vi "PWM_Lenkung_Array.vi"(7 "schräg links":dbl, 8 "schräg rechts":dbl, 9 "vorne links":dbl, 10 "vorne rechts":dbl) -> (0 "16 IR true":bool, 2 "PWM Lenkung":dbl, 3 "Linefollow_Array":bool[](array[boolean]))   [LabVIEW 2016]
doc: "VI berrechnet Abweichung des Linearray zur Mittellinie\n05.04.17_Tloe"
uses:
  <vilib>/myRIO/Instrument Drivers/Onboard IO/DIO/typedefs/DIO Reference.ctl
  <vilib>/myRIO/Common/Instrument Driver Framework/Utilities/typedefs/myRIO Generic Hardware Reference.ctl
  <vilib>/myRIO/Common/Instrument Driver Framework/Utilities/typedefs/Hardware Version Enum.ctl
  <vilib>/myRIO/Common/Instrument Driver Framework/Utilities/typedefs/myRIO v1.0 Reference.ctl
  <vilib>/myRIO/Common/Instrument Driver Framework/Utilities/typedefs/Generic FPGA Reference.ctl
  <vilib>/myRIO/Common/Instrument Driver Framework/myRIO v1.0/DIO/typedefs/DIO Channels List.ctl
  <vilib>/myRIO/Common/Instrument Driver Framework/myRIO v1.0/DIO/typedefs/DIO Channels Enum.ctl
  <vilib>/userdefined/High Color/nirio_resource_hc.ctl
  <vilib>/myRIO/Common/Instrument Driver Framework/Utilities/vis/Is FPGA Ref Available.vi
  <vilib>/myRIO/Common/Instrument Driver Framework/myRIO v1.0/DIO/vis/myRIO v1.1 Open DIO.vi
  <vilib>/myRIO/Instrument Drivers/Onboard IO/DIO/vis/Read.vi
  <vilib>/myRIO/Common/Instrument Driver Framework/Utilities/vis/Validate Channels.vi
  <vilib>/myRIO/Common/Instrument Driver Framework/myRIO v1.0/DIO/vis/myRIO v1.0 Reserve DIO.vi
  <vilib>/myRIO/Common/Instrument Driver Framework/myRIO v1.0/Resource Manager/vis/myRIO v1.0 Reserve Channel List.vi
  <vilib>/myRIO/Common/Instrument Driver Framework/myRIO v1.0/DIO/vis/myRIO v1.0 Build MUX Configuration DIO.vi
  <vilib>/myRIO/Common/Instrument Driver Framework/myRIO v1.0/Resource Manager/vis/myRIO v1.0 Reserve Channel.vi
  <vilib>/myRIO/Common/Instrument Driver Framework/myRIO v1.0/Resource Manager/vis/myRIO v1.0 Unreserve Channel.vi
  <vilib>/myRIO/Common/Instrument Driver Framework/myRIO v1.0/Resource Manager/vis/myRIO v1.0 Create Configuration List.vi
  <vilib>/myRIO/Common/Instrument Driver Framework/myRIO v1.0/Resource Manager/vis/myRIO v1.0 Build Mutex Name.vi
  <vilib>/Utility/VariantDataType/GetNumericInfo.vi
  <vilib>/Utility/error.llb/Error Cluster From Error Code.vi
  <vilib>/myRIO/Common/Instrument Driver Framework/myRIO v1.0/myRIO v1.1 Open.vi
  <vilib>/myRIO/Common/Instrument Driver Framework/Utilities/vis/IO Manager.vi
  <vilib>/myRIO/Common/Instrument Driver Framework/Utilities/vis/Configuration Manager.vi
  <vilib>/myRIO/Common/Instrument Driver Framework/myRIO v1.0/Resource Manager/vis/myRIO v1.0 Configure IO.vi
  <vilib>/myRIO/Common/Instrument Driver Framework/myRIO v1.0/myRIO v1.0 Close.vi
  <vilib>/myRIO/Common/Instrument Driver Framework/myRIO v1.0/DIO/vis/myRIO v1.0 Read DIO.vi
  <vilib>/addons/control/pid/pid.llb/PID (DBL).vi
  <vilib>/myRIO/Express VI/Onboard IO/DI/DI Express VI.xnode
  <vilib>/myRIO/Instrument Drivers/Onboard IO/DIO/vis/myRIO DIO Open.xnode
  <vilib>/myRIO/Instrument Drivers/Onboard IO/DIO/DIO.lvlib
  <vilib>/addons/control/pid/NI_PID_pid.lvlib
panel:
  in  "PID Lenkung IR":T1={"proportional gain (Kc)"=0.5, "integral time (Ti, min)"=0.0, "derivative time (Td, min)"=0.002}
  in  "PID Array":T1={"proportional gain (Kc)"=0.8, "integral time (Ti, min)"=0.08, "derivative time (Td, min)"=0.32}
  in  "Sensorarray\nZusatzwerte":dbl[](array[numeric])=[8.0, 7.0, 6.0, 5.0, 4.0, 3.0, 2.0, 1.0, -1.0, -2.0, -3.0, -4.0, -5.0, -6.0, -7.0, -8.0]
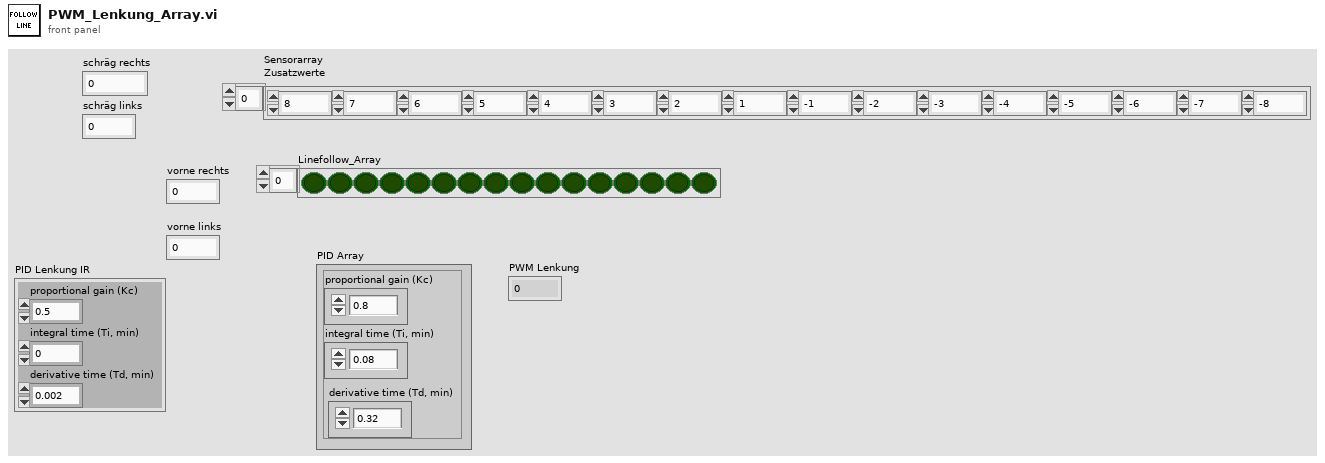
[diagram p1: front panel]
types:
  T1 = cluster{"proportional gain (Kc)":dbl, "integral time (Ti, min)":dbl, "derivative time (Td, min)":dbl}
  T2 = cluster{"A/DIO0 (Pin 11)":bool, "A/DIO1 (Pin 13)":bool, "A/DIO2 (Pin 15)":bool, "A/DIO3 (Pin 17)":bool, "A/DIO4 (Pin 19)":bool, "A/DIO5 (Pin 21)":bool, "A/DIO6 (Pin 23)":bool, "A/DIO7 (Pin 25)":bool, "B/DIO7 (Pin 25)":bool, "B/DIO6 (Pin 23)":bool, "B/DIO5 (Pin 21)":bool, "B/DIO3 (Pin 17)":bool, "B/DIO4 (Pin 19)":bool, "B/DIO2 (Pin 15)":bool, "B/DIO1 (Pin 13)":bool, "B/DIO12 (Pin 22)":bool}
  T3 = cluster{"A/DIO0 (Pin 11)":i16, "A/DIO1 (Pin 13)":i16, "A/DIO2 (Pin 15)":i16, "A/DIO3 (Pin 17)":i16, "A/DIO4 (Pin 19)":i16, "A/DIO5 (Pin 21)":i16, "A/DIO6 (Pin 23)":i16, "A/DIO7 (Pin 25)":i16, "B/DIO7 (Pin 25)":i16, "B/DIO6 (Pin 23)":i16, "B/DIO5 (Pin 21)":i16, "B/DIO3 (Pin 17)":i16, "B/DIO4 (Pin 19)":i16, "B/DIO2 (Pin 15)":i16, "B/DIO1 (Pin 13)":i16, "B/DIO12 (Pin 22)":i16}
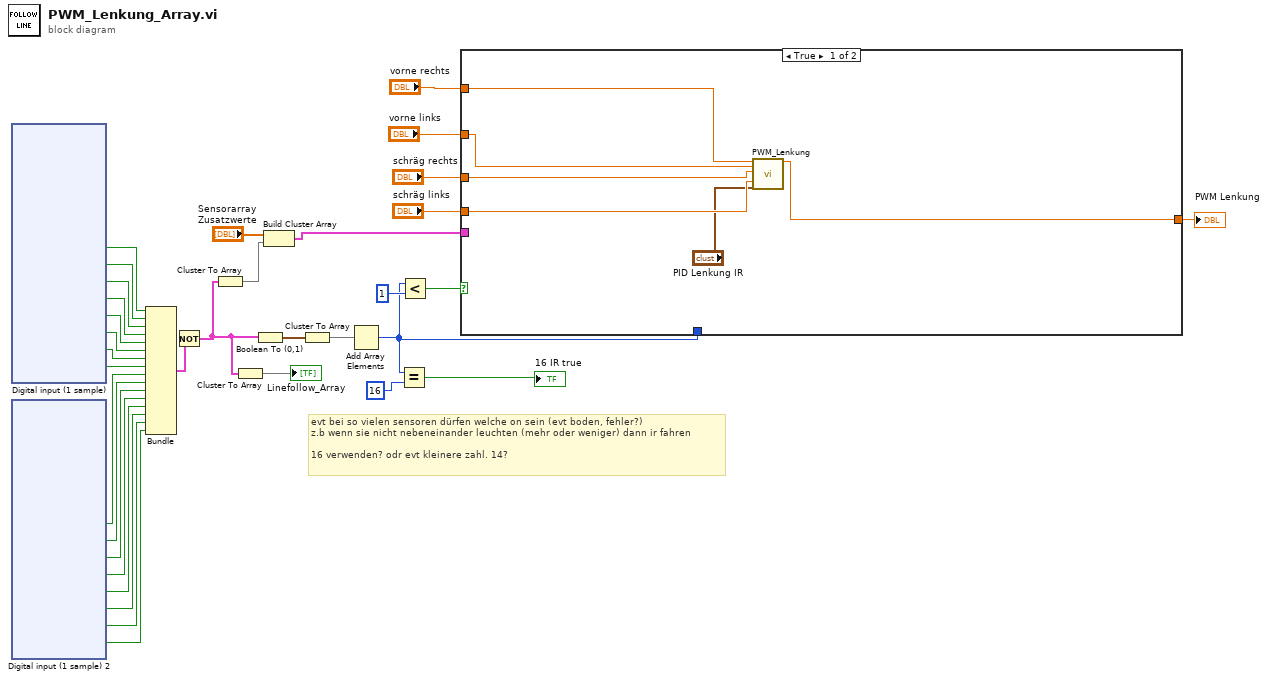
[diagram p0: block diagram]
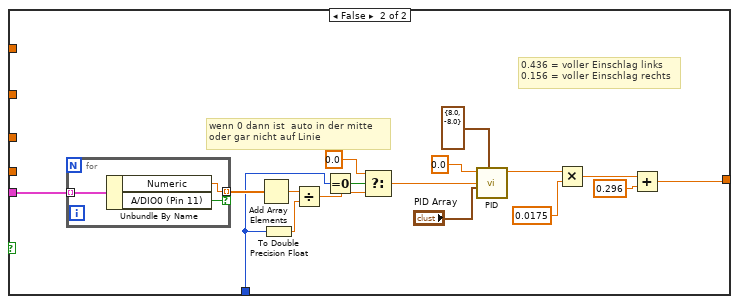
[diagram p2: hidden frame]
diagram:
  # "evt bei so vielen sensoren dürfen welche on sein (evt boden, fehler?)\nz.b wenn sie nicht nebeneinander leuchten (mehr oder weniger) dann ir fahren\n\n16 verwenden? odr evt kleinere zahl. 14?"
  n1 = xnode "Digital input (1 sample)"() -> ("A/DIO0 (Pin 11)"=w25:bool, "A/DIO1 (Pin 13)"=w26:bool, "A/DIO2 (Pin 15)"=w27:bool, "A/DIO3 (Pin 17)"=w28:bool, "A/DIO4 (Pin 19)"=w29:bool, "A/DIO5 (Pin 21)"=w30:bool, "A/DIO6 (Pin 23)"=w31:bool, "A/DIO7 (Pin 25)"=w32:bool)  [unwired: 1 in, 1 out]
  n2 = xnode "Digital input (1 sample) 2"() -> ("B/DIO7 (Pin 25)"=w10:bool, "B/DIO6 (Pin 23)"=w9:bool, "B/DIO5 (Pin 21)"=w8:bool, "B/DIO3 (Pin 17)"=w7:bool, "B/DIO4 (Pin 19)"=w6:bool, "B/DIO2 (Pin 15)"=w5:bool, "B/DIO1 (Pin 13)"=w4:bool, "B/DIO12 (Pin 22)"=w3:bool)  [unwired: 1 in, 1 out]
  n3 = Bundle("A/DIO0 (Pin 11)"=w25, "A/DIO1 (Pin 13)"=w26, "A/DIO2 (Pin 15)"=w27, "A/DIO3 (Pin 17)"=w28, "A/DIO4 (Pin 19)"=w29, "A/DIO5 (Pin 21)"=w30, "A/DIO6 (Pin 23)"=w31, "A/DIO7 (Pin 25)"=w32, "B/DIO7 (Pin 25)"=w10, "B/DIO6 (Pin 23)"=w9, "B/DIO5 (Pin 21)"=w8, "B/DIO3 (Pin 17)"=w7, "B/DIO4 (Pin 19)"=w6, "B/DIO2 (Pin 15)"=w5, "B/DIO1 (Pin 13)"=w4, "B/DIO12 (Pin 22)"=w3) -> (w24:T2)  [unwired: 1 in]
  n4 = Not(x=w24) -> (.not. x?=w17:T2)
  n5 = Cluster To Array(cluster=w17) -> (array=w19:bool[])
  n6 = Cluster To Array(cluster=w17) -> (array=→"Linefollow_Array":bool[])
  n7 = Boolean To (0,1)(Boolean=w17) -> (0, 1=w33:T3)
  n8 = Build Cluster Array("Sensorarray\nZusatzwerte", w19) -> (w14:cluster{"Numeric":dbl, "A/DIO0 (Pin 11)":bool}[])
  n9 = Cluster To Array(cluster=w33) -> (array=w16:i16[])
  n10 = Add Array Elements(numeric array=w16) -> (sum=w13:i16)
  n11 = Equal?(x=w13, y=i16 16) -> (x = y?=→"16 IR true":bool)
  n12 = Less?(x=w13, y=i16 1) -> (x < y?=w15:bool)
  n13 = case shown="True" w15 {
    tunnel: [w35 w43] -> w20
    tunnel: w14 -> [_ w42]
    tunnel: w13 -> [_ w41]
    tunnel: "vorne rechts" -> [w40 _]
    tunnel: "vorne links" -> [w39 _]
    tunnel: "schräg rechts" -> [w38 _]
    tunnel: "schräg links" -> [w37 _]
    frame True {
      n14 = call "PWM_Lenkung.vi"("vorne rechts"=w40, "vorne links"=w39, "Schräg rechts"=w38, "Schräg links"=w37, "PID gains out 2"="PID Lenkung IR") -> ("PWM Lenkung"=w35:dbl)  [unwired: 14 in]
    }
    frame False {
      # "0.436 = voller Einschlag links\n0.156 = voller Einschlag rechts"
      # "wenn 0 dann ist  auto in der mitte \noder gar nicht auf Linie"
      n15 = for {
        tunnel: [w60] -> w55 mode=indexing if=w59
        tunnel: w42 -> [w58] mode=indexing
        n16 = Unbundle By Name(w58) -> ("Numeric"=w60:dbl, "A/DIO0 (Pin 11)"=w59:bool)
      }
      n17 = Add Array Elements(numeric array=w55) -> (sum=w56:dbl)
      n18 = To Double Precision Float(number=w41) -> (double precision float=w57:dbl)
      n19 = Divide(x=w56, y=w57) -> (x/y=w54:dbl)
      n20 = Equal To 0?(x=w41) -> (x = 0?=w52:bool)
      n21 = Select(t=0.0, s=w52, f=w54) -> (s? t:f=w44:dbl)
      n22 = call-poly <vilib>:"PID.vi"("output range"=cluster{"output high":dbl, "output low":dbl} {"output high"=8.0, "output low"=-8.0}, "PID gains"="PID Array", "process variable"=w44, "setpoint"=0.0) -> ("output"=w49:dbl)  [unwired: 6 in, 1 out]
      n23 = Multiply(x=w49, y=0.0175) -> (x*y=w50:dbl)
      n24 = Add(x=w50, y=0.296) -> (x+y=w43:dbl)
    }
  }
  "PWM Lenkung" <- w20
